vi "check_instrument_error.vi"(6 "Mode (Check error from Session)":T1(ring)=enum."Check error from Session", 7 "Attribute":T2={"Identifier"="", "Descriptive name"="", "Data Type"=enum."Integer 32", "Command"="", "Access"=2, "Range Table"="", "Read Callback"="", "Write Callback"="", "Range Callback"="", "Check Callback"="", "Rngtable Callback"="", "Coerce Callback"="", "Supported Models"="", "Instrument Options"="", "Repeated Capabilities"="", "Check Status Callback"="", "Index"=0, "Flag: OPC Wait"=FALSE, "Flag: Dont check status"=FALSE, "Flag: Cache Only"=FALSE} {"Access" items=["Read Only", "Write Only", "Read/Write"]}, 8 "error in":errorcluster {"code" format="%.0x"}, 11 "VISA resource name":refnum<visa-resource-name>) -> (0 "error out":errorcluster {"code" format="%.0x"}, 3 "VISA resource name out":refnum<visa-resource-name>)   [LabVIEW 2014, in "rszvl_rsidr_core.lvlib"]
uses:
  rszvl_rsidr_core.lvlib
  type_Attribute.ctl
  type_Attribute_Data_Type.ctl
  type_Error_Codes.ctl
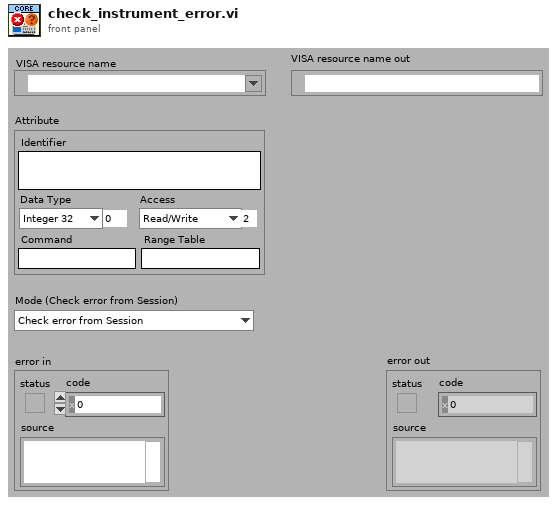
[diagram p1: front panel]
types:
  T1 = enum16{"Check error", "Don't check error", "Check error from Session"}
  T2 = typedef "rszvl_rsidr_core.lvlib/type_Attribute.ctl" = cluster{"Identifier":string, "Descriptive name":string, "Data Type":T3, "Command":string, "Access":u16, "Range Table":string, "Read Callback":string, "Write Callback":string, "Range Callback":string, "Check Callback":string, "Rngtable Callback":string, "Coerce Callback":string, "Supported Models":string, "Instrument Options":string, "Repeated Capabilities":string, "Check Status Callback":string, "Index":i32, "Flag: OPC Wait":bool, "Flag: Dont check status":bool, "Flag: Cache Only":bool}
  T3 = typedef "rszvl_rsidr_core.lvlib/type_Attribute_Data_Type.ctl" = enum16{"Integer 32", "Double", "String", "Boolean", "None", "Integer 64"}
  T4 = typedef "rszvl_rsidr_core.lvlib/type_Session_Data.ctl" = cluster{"Instr type":string, "Instr type for err. msg.":string, "Installed Options":string[], "OPC Timeout":i32, "Query Instrument Status":bool, "Check Range":bool, "Check Options":bool, "Add LF to Write":bool, "Simulate":bool, "Logging":bool, "Logging params":variant, "Interface Type":enum16{"Unknown", "GPIB", "VXI", "GPIB_VXI", "ASRL", "PXI", "TCPIP", "USB", "SOCKET"}, "Fast Sweep":i32, "AdditionalFlags":i32, "WaitBeforeWrite":i32, "WaitBeforeRead":i32, "BinDataChunkSize":i64}
  T5 = typedef "rszvl_rsidr_core.lvlib/type_Error_Codes.ctl" = enum16{"No_error", "VISA_err_ResourceNotFound", "VISA_err_Timeout", "VISA_warn_MoreDataAvailable", "RS_err_MissingCallback", "RS_err_InvalidAttribute", "RS_err_InvalidValue", "RS_err_UnknownResource", "RS_err_AlreadyInitialized", "RS_err_InstrumentStatus", "RS_err_BadRepCapName", "RS_err_TypesMismatch", "RS_err_ValueNotSupported", "RS_err_InvalidRngTable", "RS_err_IDqueryFail", "RS_err_UnexpResponse", "VISA_warn_ConfigNotLoaded", "RS_err_AttributeNotReadable", "RS_err_AttributeNotWritable", "RS_err_InstrumentType", "RS_err_InstrumentOption", "VISA_err_InvalidSize", "RS_err_ReliabilityIndicator", "VISA_warn_UnknownStatus", "VISA_warn_TermCharRead", "VISA_err_IO_error"}
  T6 = enum16{"Unknown", "GPIB", "VXI", "GPIB_VXI", "ASRL", "PXI", "TCPIP", "USB", "SOCKET"}
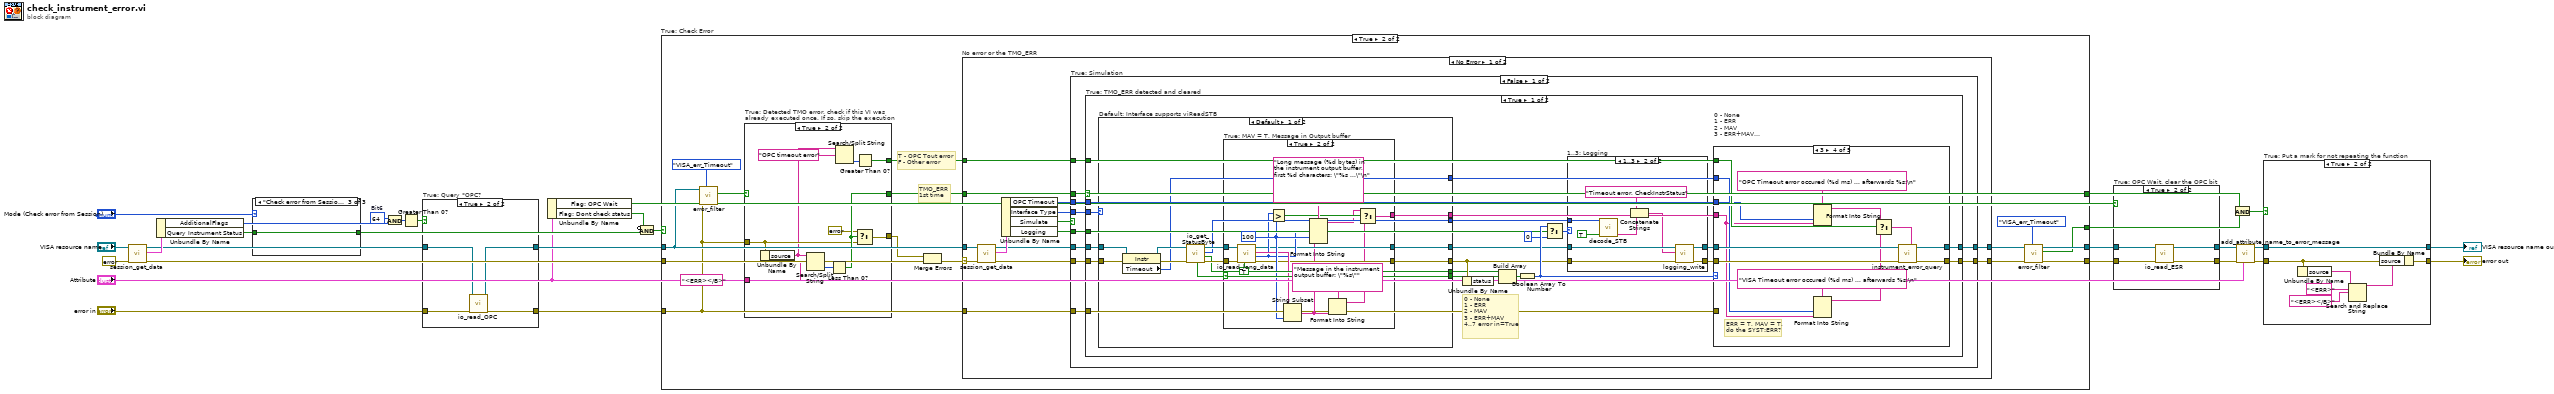
[diagram p0: block diagram]
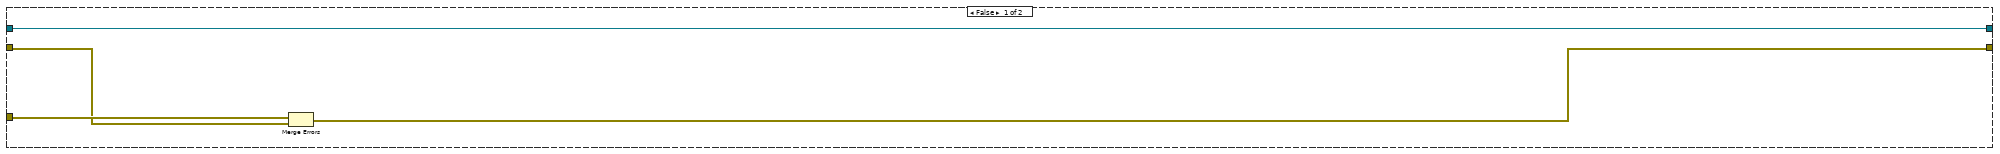
[diagram p5: hidden frame]
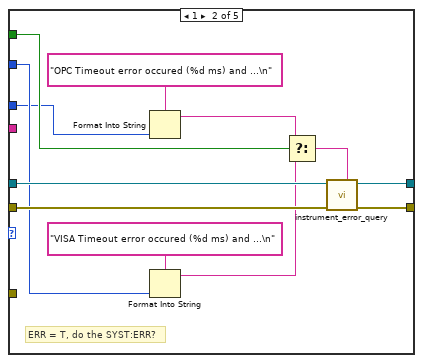
[diagram p8: hidden frame]
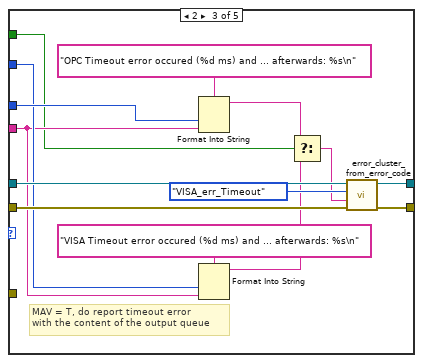
[diagram p9: hidden frame]
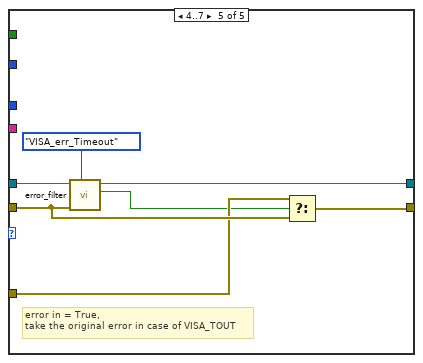
[diagram p10: hidden frame]
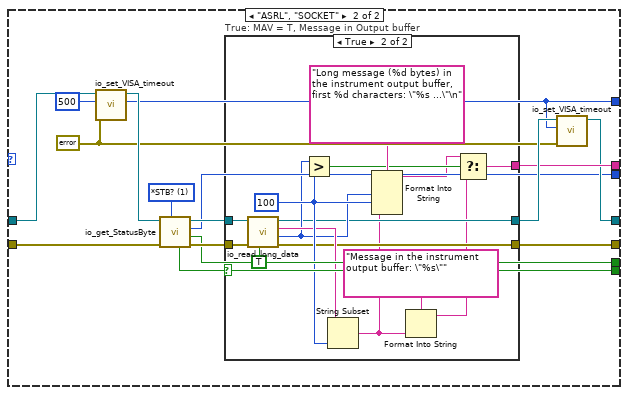
[diagram p13: hidden frame]
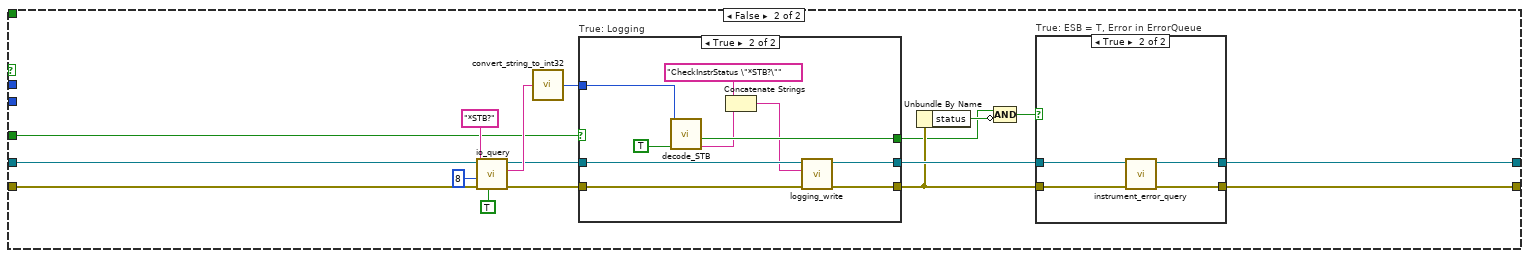
[diagram p15: hidden frame]
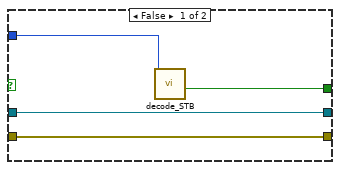
[diagram p17: hidden frame]
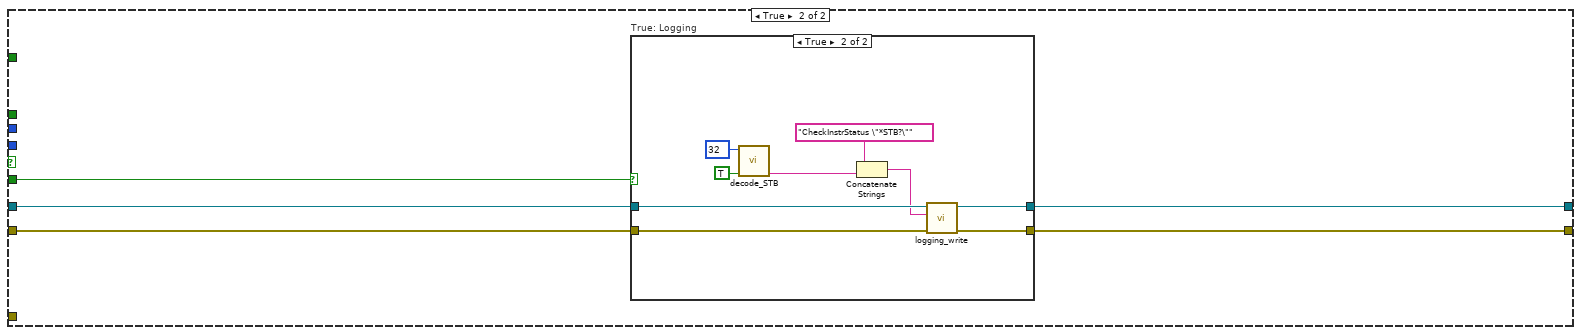
[diagram p18: hidden frame]
diagram:
  w17 = 64  # Bit6
  n1 = call "session_get_data.vi"("error in"=errorcluster {"status"=FALSE, "code"=0, "source"=""}, "VISA resource name"="VISA resource name") -> ("error out"=w12:errorcluster, "Session User Data out"=w21:T4, "VISA resource name out"=w14:refnum<visa-resource-name>)  [unwired: 7 in]
  n2 = Unbundle By Name(w21) -> ("AdditionalFlags"=w18:i32, "Query Instrument Status"=w19:bool)
  n3 = case shown="\"Check error from Session\"" "Mode (Check error from Session)" {
    tunnel: [TRUE ("Boolean Out") _ w31] -> w28
    tunnel: w19 -> [_ _ w31]
    frame "Check error" {
    }
    frame "Don't check error" {
    }
    frame "Check error from Session" {
    }
  }
  n4 = And(x=w17, y=w18) -> (x .and. y?=w16:i32)
  n5 = Greater Than 0?(x=w16) -> (x > 0?=w15:bool)
  n6 = case "True: Query *OPC?" shown="True" w15 {
    tunnel: w14 -> [w32 w35]
    tunnel: [w32 w34] -> w13
    tunnel: "error in" -> [w33 w37]
    tunnel: [w33 w36] -> w10
    frame False {
    }
    frame True {
      n7 = call "io_read_OPC.vi"("error in"=w37, "VISA resource name"=w35) -> ("error out"=w36:errorcluster, "VISA resource name out"=w34:refnum<visa-resource-name>)  [unwired: 7 in, 1 out]
    }
  }
  n8 = Unbundle By Name("Attribute") -> ("Flag: OPC Wait"=w26:bool, "Flag: Dont check status"=w23:bool)
  n9 = Compound Arithmetic op=AND(invert w23, w28) -> (w27:bool)
  n10 = case "True: Check Error" shown="True" w27 {
    tunnel: [w41 w44] -> w24
    tunnel: [w39 w45] -> w25
    tunnel: w13 -> [w41 w55]
    tunnel: w12 -> [w38 w56]
    tunnel: w10 -> [w40 w52]
    tunnel: [_ w49] -> w2
    tunnel: [_ w43] -> w1
    frame False {
      n11 = Merge Errors(w40, w38) -> (w39:errorcluster)
    }
    frame True {
      # "T - OPC Tout error\nF - Other error"
      # "TMO_ERR\n1st time"
      n12 = call "error_filter.vi"("Error Enum in"=type_Error_Codes."VISA_err_Timeout", "error in"=w52, "VISA resource name"=w55) -> ("Code Detected"=w53:bool)  [unwired: 6 in, 2 out]
      n13 = case "True: Detected TMO error, check if this VI was\nalready executed once. If so, skip the execution" shown="True" w53 {
        tunnel: w52 -> [w58 w65]
        tunnel: [w58 w67] -> w51
        tunnel: [_ w66] -> w49
        tunnel: "<ERR></B>" ("search string/char (-)") -> [_ w63]
        tunnel: [_ w61] -> w42
        frame False {
        }
        frame True {
          n14 = Unbundle By Name(w65) -> ("source"=w60:string)
          n15 = Search/Split String(string=w60, search string/char (-)=w63) -> (offset of match=w68:i32)  [unwired: 1 in, 2 out]
          n16 = Less Than 0?(x=w68) -> (x < 0?=w66:bool)
          n17 = Search/Split String(string=w60, search string/char (-)="OPC timeout error") -> (offset of match=w62:i32)  [unwired: 1 in, 2 out]
          n18 = Select(t=errorcluster {"status"=FALSE, "code"=0, "source"=""} ("f"), s=w66, f=w65) -> (s? t:f=w67:errorcluster)
          n19 = Greater Than 0?(x=w62) -> (x > 0?=w61:bool)
        }
      }
      n20 = Merge Errors(w51, w56) -> (w54:errorcluster)
      n21 = case "No error or the TMO_ERR" shown="No Error" w54 {
        selector: w54 -> [w76 w291]
        tunnel: [w81 w292] -> w46
        tunnel: [w82 w291] -> w47
        tunnel: w55 -> [w80 w292]
        tunnel: w49 -> [w75 _]
        tunnel: w52 -> [w73 _]
        tunnel: w42 -> [w69 _]
        frame No Error {
          n22 = call "session_get_data.vi"("error in"=w76, "VISA resource name"=w80) -> ("error out"=w78:errorcluster, "Session User Data out"=w79:T4, "VISA resource name out"=w77:refnum<visa-resource-name>)  [unwired: 7 in]
          n23 = Unbundle By Name(w79) -> ("OPC Timeout"=w70:i32, "Interface Type"=w74:T6, "Simulate"=w72:bool, "Logging"=w71:bool)
          n24 = case "True: Simulation" shown="False" w72 {
            tunnel: [w87 w277] -> w82
            tunnel: [w88 w276] -> w81
            tunnel: w78 -> [w91 w279]
            tunnel: w77 -> [w92 w278]
            tunnel: w75 -> [w90 _]
            tunnel: w74 -> [w89 _]
            tunnel: w73 -> [w86 _]
            tunnel: w71 -> [w85 w275]
            tunnel: w70 -> [w84 _]
            tunnel: w69 -> [w83 _]
            frame False {
              n25 = case "True: TMO_ERR detected and cleared" shown="True" w90 {
                tunnel: w92 -> [w102 w250]
                tunnel: w91 -> [w101 w249]
                tunnel: [w98 w244] -> w88
                tunnel: [w97 w243] -> w87
                tunnel: w89 -> [w100 _]
                tunnel: w86 -> [w95 _]
                tunnel: w85 -> [w96 w238]
                tunnel: w84 -> [w94 _]
                tunnel: w83 -> [w93 _]
                frame True {
                  # "0 - None\n1 - ERR\n2 - MAV\n3 - ERR+MAV\n4..7 error in=True"
                  n26 = case "Default: Interface supports viReadSTB" shown="Default" w100 {
                    tunnel: w102 -> [w177 w218]
                    tunnel: w101 -> [w179 w213]
                    tunnel: [w185 w211] -> w109
                    tunnel: [w183 w208] -> w107
                    tunnel: [w184 w210] -> w106
                    tunnel: [w182 w209] -> w112
                    tunnel: [w181 w207] -> w110
                    tunnel: [w180 w206] -> w111
                    tunnel: [w175 w205] -> w99
                    frame Default {
                      n27 = property on="Property Node" class="Instr"(reference=w177, error in=w179) -> (reference out=w176:refnum<visa-resource-name>, error out=w178:errorcluster, "Timeout"=w175:u32)
                      n28 = call "io_get_StatusByte.vi"("error in"=w178, "VISA resource name"=w176) -> ("error out"=w186:errorcluster, "Error"=w184:bool, "STB returned"=w180:u16, "VISA resource name out"=w187:refnum<visa-resource-name>, "MAV"=w183:bool)  [unwired: 4 in, 1 out]
                      n29 = case "True: MAV = T, Message in Output buffer" shown="True" w183 {
                        tunnel: w186 -> [w189 w204]
                        tunnel: w187 -> [w188 w202]
                        tunnel: [w189 w197] -> w185
                        tunnel: [w188 w198] -> w181
                        tunnel: [_ w190] -> w182
                        frame False {
                        }
                        frame True {
                          w201 = u32 100 ("y")
                          n30 = call "io_read_long_data.vi"("Block Logging (F)"=TRUE, "error in"=w204, "VISA resource name"=w202) -> ("error out"=w197:errorcluster, "return count"=w199:u32, "read buffer"=w200:string, "VISA resource name out"=w198:refnum<visa-resource-name>)  [unwired: 5 in]
                          n31 = Greater?(x=w199, y=w201) -> (0:w193:bool)
                          n32 = String Subset(string=w200, length (rest)=w201) -> (substring=w195:string)  [unwired: 1 in]
                          n33 = Format Into String(format string="Long message (%d bytes) in the instrument output buffer, first %d characters: \"%s ...\"\n", w199, w201, w195) -> (resulting string=w192:string)  [unwired: 2 in, 1 out]
                          n34 = Format Into String(format string="Message in the instrument output buffer: \"%s\"", w195) -> (resulting string=w191:string)  [unwired: 2 in, 1 out]
                          n35 = Select(t=w192, s=w193, f=w191) -> (s? t:f=w190:string)
                        }
                      }
                    }
                    frame "ASRL", "SOCKET" {
                      w212 = errorcluster {"status"=FALSE, "code"=0, "source"=""} ("error in")
                      w215 = u16 1 items=["viReadSTB", "*STB?"] ("Method (viReadSTB)")
                      n36 = call "io_set_VISA_timeout.vi"("error in"=w212, "VISA Timeout"=u32 500, "VISA resource name"=w218) -> ("Old VISA Timeout"=w205:u32, "VISA resource name out"=w217:refnum<visa-resource-name>)  [unwired: 6 in, 1 out]
                      n37 = call "io_get_StatusByte.vi"("Method (viReadSTB)"=w215, "error in"=w213, "VISA resource name"=w217) -> ("error out"=w220:errorcluster, "Error"=w210:bool, "STB returned"=w206:u16, "VISA resource name out"=w219:refnum<visa-resource-name>, "MAV"=w208:bool)  [unwired: 3 in, 1 out]
                      n38 = case "True: MAV = T, Message in Output buffer" shown="True" w208 {
                        tunnel: w220 -> [w222 w237]
                        tunnel: w219 -> [w221 w235]
                        tunnel: [w222 w230] -> w211
                        tunnel: [w221 w231] -> w214
                        tunnel: [_ w223] -> w209
                        frame False {
                        }
                        frame True {
                          w234 = u32 100 ("y")
                          n39 = call "io_read_long_data.vi"("Block Logging (F)"=TRUE, "error in"=w237, "VISA resource name"=w235) -> ("error out"=w230:errorcluster, "return count"=w232:u32, "read buffer"=w233:string, "VISA resource name out"=w231:refnum<visa-resource-name>)  [unwired: 5 in]
                          n40 = Greater?(x=w232, y=w234) -> (0:w226:bool)
                          n41 = String Subset(string=w233, length (rest)=w234) -> (substring=w228:string)  [unwired: 1 in]
                          n42 = Format Into String(format string="Long message (%d bytes) in the instrument output buffer, first %d characters: \"%s ...\"\n", w232, w234, w228) -> (resulting string=w225:string)  [unwired: 2 in, 1 out]
                          n43 = Format Into String(format string="Message in the instrument output buffer: \"%s\"", w228) -> (resulting string=w224:string)  [unwired: 2 in, 1 out]
                          n44 = Select(t=w225, s=w226, f=w224) -> (s? t:f=w223:string)
                        }
                      }
                      n45 = call "io_set_VISA_timeout.vi"("error in"=w212, "VISA Timeout"=w205, "VISA resource name"=w214) -> ("VISA resource name out"=w207:refnum<visa-resource-name>)  [unwired: 6 in, 2 out]
                    }
                  }
                  n46 = Unbundle By Name(w109) -> ("status"=w105:bool)
                  n47 = Build Array(w106, w107, w105) -> (w104:bool[])
                  n48 = Boolean Array To Number(Boolean array=w104) -> (number=w115:u32)
                  n49 = Select(t=w115, s=w96, f=u32 0) -> (s? t:f=w108:u32)
                  n50 = case "1..3: Logging" shown="1..3" w108 {
                    tunnel: w109 -> [w165 w173]
                    tunnel: [w165 w172] -> w114
                    tunnel: [w164 w171] -> w113
                    tunnel: w110 -> [w164 w170]
                    tunnel: w111 -> [_ w167]
                    frame Default {
                    }
                    frame 1..3 {
                      n51 = call "decode_STB.vi"("Compose Summary String  (F)"=TRUE, "STB in"=w167) -> ("Summary string"=w166:string)  [unwired: 6 in, 3 out]
                      n52 = Concatenate Strings("Timeout error, CheckInstrStatus" ("String to write"), w166) -> (w168:string)
                      n53 = call "logging_write.vi"("error in"=w173, "String to write"=w168, "VISA resource name"=w170) -> ("error out"=w172:errorcluster, "VISA resource name out"=w171:refnum<visa-resource-name>)  [unwired: 7 in]
                    }
                  }
                  n54 = case "0 - None\n1 - ERR\n2 - MAV\n3 - ERR+MAV\n4..7 error in=True" shown="3" w115 {
                    tunnel: w95 -> [w116 _ _ _ w158]
                    tunnel: [w116 w129 w139 w156 w160] -> w97
                    tunnel: w113 -> [w117 w126 w141 w153 w162]
                    tunnel: [w117 w128 w143 w155 w161] -> w98
                    tunnel: w114 -> [_ w125 w140 w152 w159]
                    tunnel: w112 -> [_ _ w134 w144 _]
                    tunnel: w99 -> [_ w124 w135 w151 _]
                    tunnel: w94 -> [_ w121 w137 w148 _]
                    tunnel: w93 -> [_ w123 w131 w150 _]
                    frame 0, Default {
                      # "ERR = F, MAV = F, pass the TMO_ERR forward"
                    }
                    frame 1 {
                      # "ERR = T, do the SYST:ERR?"
                      n55 = Format Into String(format string="OPC Timeout error occured (%d ms) and ...\n" ("Beginning error message string (\"\")"), w121) -> (resulting string=w120:string)  [unwired: 2 in, 1 out]
                      n56 = Format Into String(format string="VISA Timeout error occured (%d ms) and ...\n" ("Beginning error message string (\"\")"), w124) -> (resulting string=w119:string)  [unwired: 2 in, 1 out]
                      n57 = Select(t=w120, s=w123, f=w119) -> (s? t:f=w118:string)
                      n58 = call "instrument_error_query.vi"("Beginning error message string (\"\")"=w118, "error in"=w125, "VISA resource name"=w126) -> ("error out"=w129:errorcluster, "VISA resource name out"=w128:refnum<visa-resource-name>)  [unwired: 5 in, 2 out]
                    }
                    frame 2 {
                      # "MAV = T, do report timeout error\nwith the content of the output queue"
                      n59 = Format Into String(format string="OPC Timeout error occured (%d ms) and ... afterwards: %s\n" ("Beginning error message string (\"\")"), w137, w134) -> (resulting string=w133:string)  [unwired: 2 in, 1 out]
                      n60 = Format Into String(format string="VISA Timeout error occured (%d ms) and ... afterwards: %s\n" ("Beginning error message string (\"\")"), w135, w134) -> (resulting string=w132:string)  [unwired: 2 in, 1 out]
                      n61 = Select(t=w133, s=w131, f=w132) -> (s? t:f=w130:string)
                      n62 = call "error_cluster_from_error_code.vi"("error in"=w140, "error message (\"\")"=w130, "Error Enum in"=type_Error_Codes."VISA_err_Timeout", "VISA resource name"=w141) -> ("error out"=w139:errorcluster, "VISA resource name out"=w143:refnum<visa-resource-name>)  [unwired: 6 in]
                    }
                    frame 3 {
                      # "ERR = T, MAV = T,\ndo the SYST:ERR?"
                      n63 = Format Into String(format string="OPC Timeout error occured (%d ms) ... afterwards %s:\n" ("Beginning error message string (\"\")"), w148, w144) -> (resulting string=w147:string)  [unwired: 2 in, 1 out]
                      n64 = Format Into String(format string="VISA Timeout error occured (%d ms) ... afterwards %s:\n" ("Beginning error message string (\"\")"), w151, w144) -> (resulting string=w146:string)  [unwired: 2 in, 1 out]
                      n65 = Select(t=w147, s=w150, f=w146) -> (s? t:f=w145:string)
                      n66 = call "instrument_error_query.vi"("Beginning error message string (\"\")"=w145, "error in"=w152, "VISA resource name"=w153) -> ("error out"=w156:errorcluster, "VISA resource name out"=w155:refnum<visa-resource-name>)  [unwired: 5 in, 2 out]
                    }
                    frame 4..7 {
                      # "error in = True,\ntake the original error in case of VISA_TOUT"
                      n67 = call "error_filter.vi"("Error Enum in"=type_Error_Codes."VISA_err_Timeout", "error in"=w159, "VISA resource name"=w162) -> ("Code Detected"=w157:bool, "VISA resource name out"=w161:refnum<visa-resource-name>)  [unwired: 6 in, 1 out]
                      n68 = Select(t=w158, s=w157, f=w159) -> (s? t:f=w160:errorcluster)
                    }
                  }
                }
                frame False {
                  n69 = call "io_query.vi"("Block Logging (F)"=TRUE, "error in"=w249, "Bytes to read (2048)"=u32 8 ("byte count (0)"), "write buffer"="*STB?" ("write buffer (\"\")"), "VISA resource name"=w250) -> ("error out"=w246:errorcluster, "read buffer"=w252:string, "VISA resource name out"=w247:refnum<visa-resource-name>)  [unwired: 3 in, 1 out]
                  n70 = call "convert_string_to_int32.vi"("String in"=w252) -> ("int32 value out"=w248:i32)  [unwired: 4 in]
                  n71 = case "True: Logging" shown="True" w238 {
                    tunnel: w246 -> [w263 w273]
                    tunnel: [w263 w272] -> w242
                    tunnel: [w262 w271] -> w245
                    tunnel: w247 -> [w262 w270]
                    tunnel: [w264 w269] -> w240
                    tunnel: w248 -> [w261 w266]
                    frame False {
                      n72 = call "decode_STB.vi"("STB in"=w261) -> ("Error"=w264:bool)  [unwired: 7 in, 3 out]
                    }
                    frame True {
                      n73 = call "decode_STB.vi"("Compose Summary String  (F)"=TRUE, "STB in"=w266) -> ("Summary string"=w265:string, "Error"=w269:bool)  [unwired: 6 in, 2 out]
                      n74 = Concatenate Strings("CheckInstrStatus \"*STB?\"" ("String to write"), w265) -> (w267:string)
                      n75 = call "logging_write.vi"("error in"=w273, "String to write"=w267, "VISA resource name"=w270) -> ("error out"=w272:errorcluster, "VISA resource name out"=w271:refnum<visa-resource-name>)  [unwired: 7 in]
                    }
                  }
                  n76 = Unbundle By Name(w242) -> ("status"=w241:bool)
                  n77 = Compound Arithmetic op=AND(w240, invert w241) -> (w239:bool)
                  n78 = case "True: ESB = T, Error in ErrorQueue" shown="True" w239 {
                    tunnel: [w255 w260] -> w243
                    tunnel: [w256 w259] -> w244
                    tunnel: w242 -> [w255 w258]
                    tunnel: w245 -> [w256 w257]
                    frame False {
                    }
                    frame True {
                      n79 = call "instrument_error_query.vi"("error in"=w258, "VISA resource name"=w257) -> ("error out"=w260:errorcluster, "VISA resource name out"=w259:refnum<visa-resource-name>)  [unwired: 6 in, 2 out]
                    }
                  }
                }
              }
            }
            frame True {
              n80 = case "True: Logging" shown="True" w275 {
                tunnel: w279 -> [w281 w290]
                tunnel: w278 -> [w280 w289]
                tunnel: [w281 w288] -> w277
                tunnel: [w280 w287] -> w276
                frame False {
                }
                frame True {
                  n81 = call "decode_STB.vi"("Compose Summary String  (F)"=TRUE, "STB in"=32) -> ("Summary string"=w282:string)  [unwired: 6 in, 3 out]
                  n82 = Concatenate Strings("CheckInstrStatus \"*STB?\"" ("String to write"), w282) -> (w283:string)
                  n83 = call "logging_write.vi"("error in"=w290, "String to write"=w283, "VISA resource name"=w289) -> ("error out"=w288:errorcluster, "VISA resource name out"=w287:refnum<visa-resource-name>)  [unwired: 7 in]
                }
              }
            }
          }
        }
        frame Error {
          # "Communication error or error\nchecking turned off"
        }
      }
      n84 = call "error_filter.vi"("Error Enum in"=type_Error_Codes."VISA_err_Timeout", "error in"=w47, "VISA resource name"=w46) -> ("error out"=w45:errorcluster, "Code Detected"=w43:bool, "VISA resource name out"=w44:refnum<visa-resource-name>)  [unwired: 6 in]
    }
  }
  n85 = case "True: OPC Wait, clear the OPC bit" shown="True" w26 {
    tunnel: w25 -> [w294 w298]
    tunnel: w24 -> [w293 w297]
    tunnel: [w294 w296] -> w6
    tunnel: [w293 w295] -> w9
    frame False {
    }
    frame True {
      n86 = call "io_read_ESR.vi"("error in"=w298, "VISA resource name"=w297) -> ("error out"=w296:errorcluster, "VISA resource name out"=w295:refnum<visa-resource-name>)  [unwired: 7 in, 1 out]
    }
  }
  n87 = And(x=w2, y=w1) -> (x .and. y?=w4:bool)
  n88 = call "add_attribute_name_to_error_message.vi"("Attribute"="Attribute", "error in"=w6) -> ("error out"=w5:errorcluster)  [unwired: 8 in, 1 out]
  n89 = case "True: Put a mark for not repeating the function" shown="True" w4 {
    tunnel: w5 -> [w300 w302]
    tunnel: w9 -> [w299 w304]
    tunnel: [w299 w304] -> w8
    tunnel: [w300 w303] -> w7
    frame False {
    }
    frame True {
      n90 = Unbundle By Name(w302) -> ("source"=w306:string)
      n91 = Search and Replace String(input string=w306, search string="<ERR>", replace string="<ERR></B>" ("replace string (\"\")")) -> (result string=w301:string)  [unwired: 5 in, 3 out]
      n92 = Bundle By Name(cluster=w302, "source"=w301) -> (w303:errorcluster)
    }
  }
  "error out" <- w7
  "VISA resource name out" <- w8
